vi "pr1.vi"() -> ()   [LabVIEW 2014]
uses:
  <vilib>/measure/NI_MABase.lvlib
panel:
  in  "L":dbl(slide)=2e-06 min=1e-06 max=0.001 step=1e-07 scale=1e-06..0.001 scale format="%#.6p"
  in  "DutyCycle":dbl(slide)=50.0 caption="Duty Cycle (%)" min=0.0 max=100.0 step=1.0 scale=0.0..100.0 scale format="%#.6p"
  in  "Frequency":dbl(slide)=50.0 caption="Signal Frequency (Hz)" min=0.0 max=500.0 step=1.0 scale=0.0..100.0 scale format="%#.6p"
  in  "V":dbl(slide)=10.0 caption="Signal Voltage (V)" min=0.0 max=20.0 step=0.1 scale=0.0..20.0 scale format="%#.6p"
  in  "C":dbl(slide)=2e-06 min=1e-06 max=0.001 step=1e-07 scale=1e-06..0.001 scale format="%#.6p"
  in  "R":dbl(slide)=500.0 min=10.0 max=100000.0 step=1.0 scale=10.0..100000.0 scale format="%#.6p"
  out "Control Signal":waveform(dbl)[](graph)
  in  "stop":bool
  # "PSI3214"
  # "Laboratório de \nInstrumentação Elétrica"
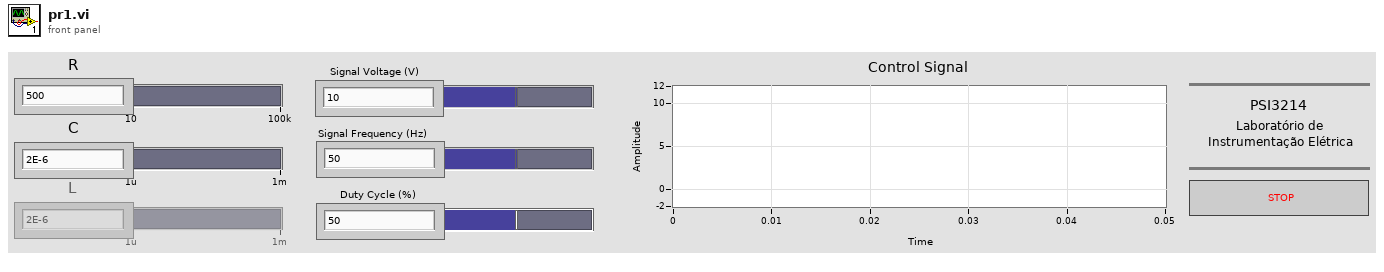
[diagram p1: front panel]
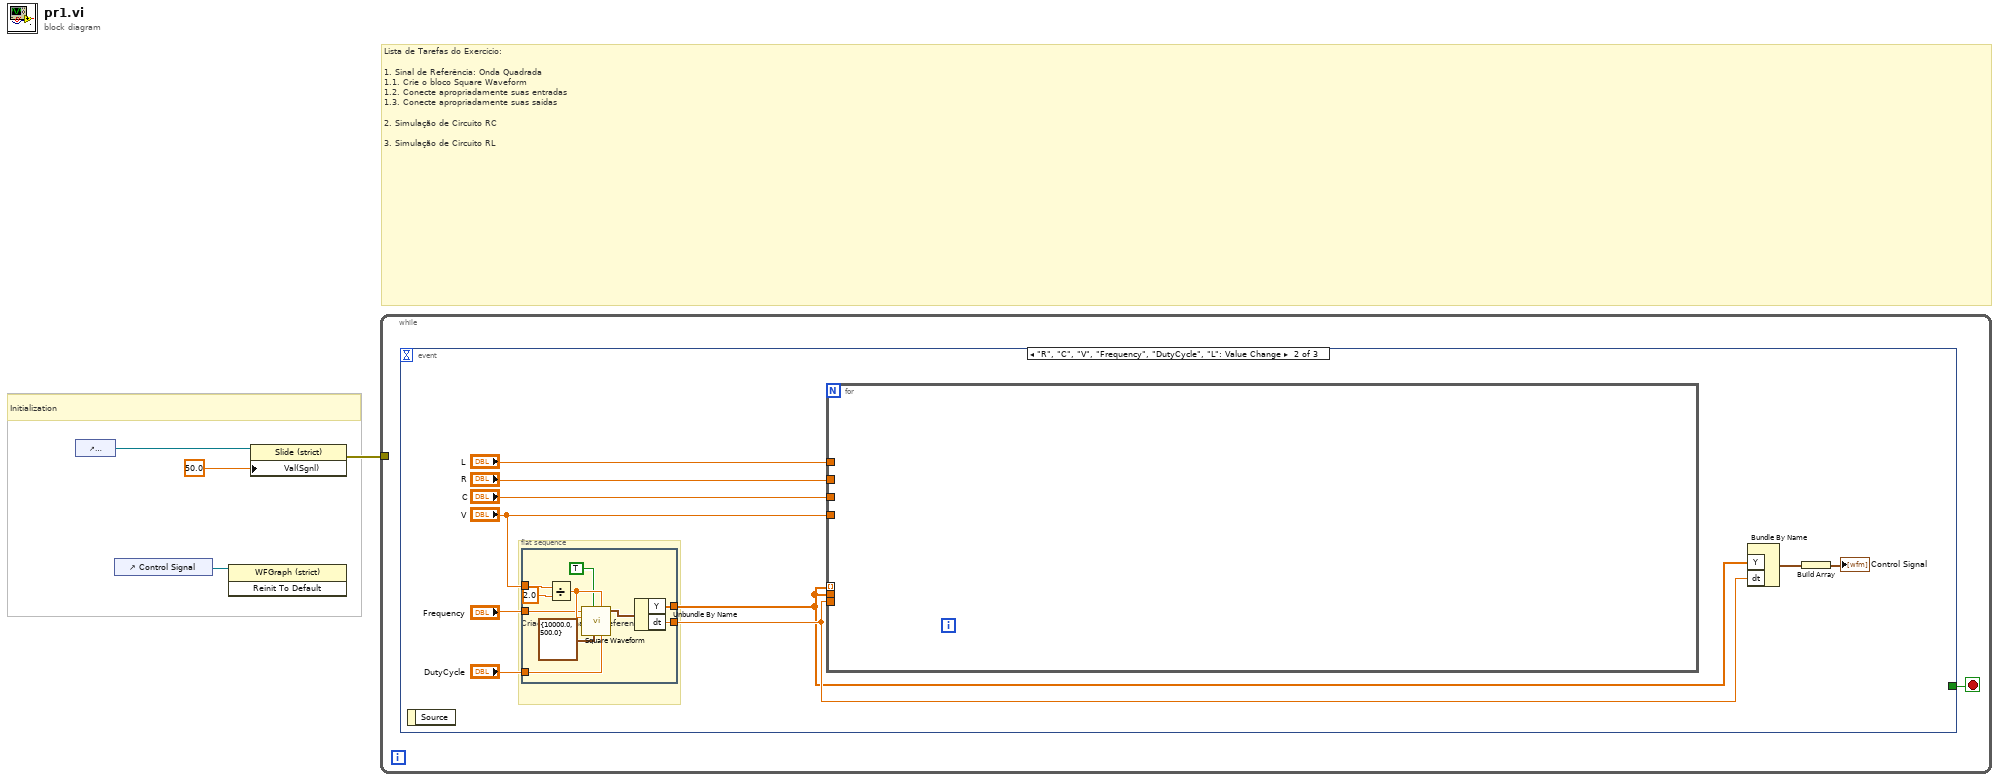
[diagram p0: block diagram]
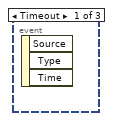
[diagram p2: hidden frame]
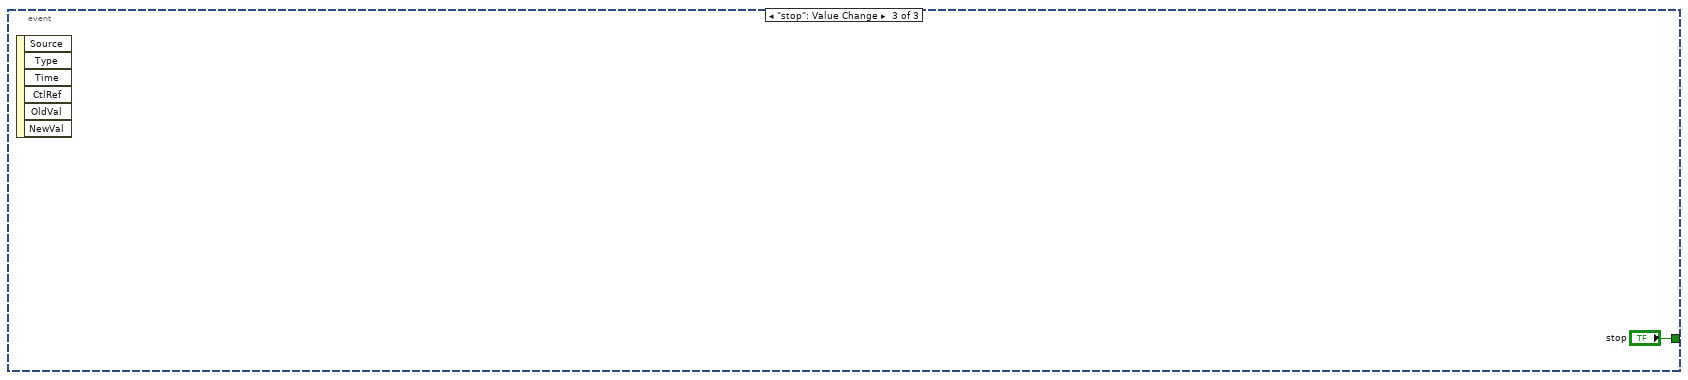
[diagram p3: hidden frame]
diagram:
  # "Initialization"
  # "Lista de Tarefas do Exercício:\n\n1. Sinal de Referência: Onda Quadrada\n1.1. Crie o bloco Square Waveform\n1.2. Conecte apropriadamente suas entradas\n1.3. Conecte apropriadamente suas saídas\n\n2. Simulação de Circuito RC\n\n3. Simulação de Circuito RL"
  n1 = control-ref of="Frequency"() -> (w1:refnum<vi>)
  n2 = control-ref of="Control Signal"() -> (w2:refnum<vi>)
  n3 = invoke class="WFGraph (strict)" method="Reinit To Default"(reference=w2) -> ()  [unwired: 2 in, 3 out]
  n4 = property class="Slide (strict)"(reference=w1, "Val(Sgnl)"=50.0 ("Value (Signaling)")) -> (error out=w3:errorcluster)  [unwired: 1 in, 1 out]
  n5 = while {
    tunnel: w3 -> [_]
    stop <- w5 stop-if-true
    n6 = event shown="[1] \"R\", \"C\", \"V\", \"Frequency\", \"DutyCycle\", \"L\": Value Change" {
      selector: _ -> [_ _ _]
      dyn-events: _ -> [_ _ _]
      timeout: _ -> [_ _ _]
      tunnel: [_ _ "stop"] -> w5
      event Timeout {
        n7 = event-data() -> ()  [unwired: 1 in, 3 out]
      }
      event "R", "C", "V", "Frequency", "DutyCycle", "L": Value Change {
        # "Criação do Sinal de Referencia"
        n8 = event-data() -> ()  [unwired: 1 in, 1 out]
        n9 = flat-sequence {
          tunnel: "V" -> [w23]
          tunnel: "Frequency" -> [w20]
          tunnel: "DutyCycle" -> [w19]
          tunnel: [w25] -> w13
          tunnel: [w24] -> w12
          frame #0 {
            n10 = Divide(x=w23, y=2.0) -> (x/y=w22:dbl)
            n11 = call <vilib>:"Square Waveform.vi"("duty cycle (%)"=w19, "offset"=w22, "sampling info"=cluster{"Fs":dbl, "#s":dbl} {"Fs"=10000.0, "#s"=500.0}, "reset signal"=TRUE, "amplitude"=w22, "frequency"=w20) -> ("signal out"=w16:waveform(dbl))  [unwired: 4 in, 1 out]
            n12 = Unbundle By Name(w16) -> ("Y"=w24:dbl[], "dt"=w25:dbl)
          }
        }
        n13 = for {
          tunnel: "R" -> [_]
          tunnel: "C" -> [_]
          tunnel: "V" -> [_]
          tunnel: w12 -> [_] mode=indexing
          tunnel: w12 -> [_]
          tunnel: w13 -> [_]
          tunnel: "L" -> [_]
        }
        n14 = Bundle By Name("Y"=w12, "dt"=w13) -> (w15:waveform(dbl))  [unwired: 1 in]
        n15 = Build Array(w15) -> (→"Control Signal":waveform(dbl)[])
      }
      event "stop": Value Change {
        n16 = event-data() -> ()  [unwired: 1 in, 6 out]
      }
    }
  }
